vi "Joysticks to Drive Motors.vi"(8 "Boost?":bool, 9 "Turn":dbl, 10 "Throttle":dbl) -> (2 "Drive Motor Values":cluster{"Left Motor":dbl, "Right Motor":dbl})   [LabVIEW 2018]
uses:
  Robot Global Data.vi
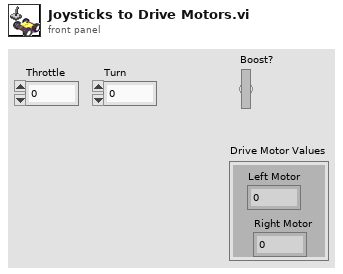
[diagram p1: front panel]
types:
  T1 = cluster{"Left Motor Value":dbl, "Right Motor Value":dbl}
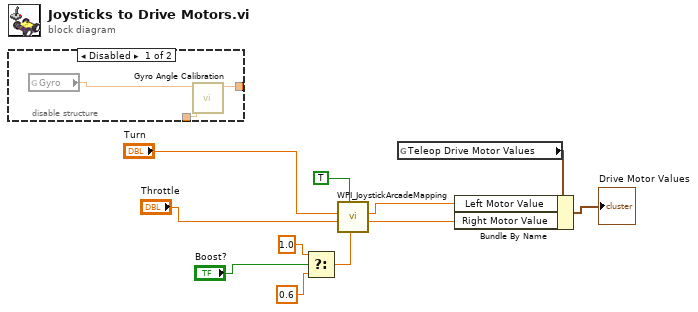
[diagram p0: block diagram]
diagram:
  n1 = disable-structure shown="Disabled" {
    disable-tunnel: _ -> [w14 _]
    disable-tunnel: [w13 _] -> _
    frame Disabled {
      n2 = global read "Robot Global Data.vi" "Gyro"() -> (w12:dbl)
      n3 = call "Gyro Angle Calibration.vi"("turning joystick input"=w14, "Gyro"=w12) -> ("adjusted turning output"=w13:dbl)  [unwired: 9 in]
    }
    frame Enabled {
    }
  }
  n4 = Select(t=1.0 ("Max Output"), s="Boost?", f=0.6 ("Max Output")) -> (s? t:f=w11:dbl)
  n5 = call <vilib>:"WPI_JoystickArcadeMapping.vi"("Max Output"=w11, "Square Inputs"=TRUE, "Y axis value"="Throttle", "X axis value"="Turn") -> ("Right Motor Value"=w3:dbl, "Left Motor Value"=w4:dbl)  [unwired: 6 in]
  n6 = global read "Robot Global Data.vi" "Teleop Drive Motor Values"() -> (w5:T1)
  n7 = Bundle By Name(cluster=w5, "Left Motor Value"=w4, "Right Motor Value"=w3) -> (→"Drive Motor Values":T1)
